vi "Integral.vi"(5 "End":dbl, 7 "Start":dbl, 11 "Spectras-Analiza":cluster{dbl[], dbl[]}[](array[cluster])) -> (3 "Integral":dbl[](array[numeric]))   [LabVIEW 2020]
uses:
  <vilib>/Analysis/2dsp.llb/Integral Method.ctl
  <vilib>/Analysis/8numeric.llb/1D Numeric Integration.vi
  <vilib>/Analysis/NI_AALPro.lvlib
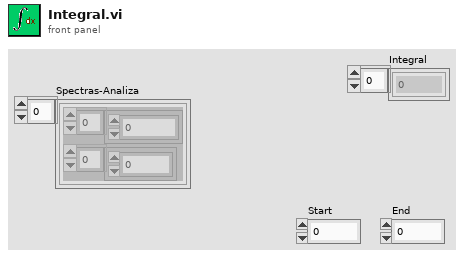
[diagram p1: front panel]
types:
  T1 = typedef "NI_AALPro.lvlib/Integral Method.ctl" = i32
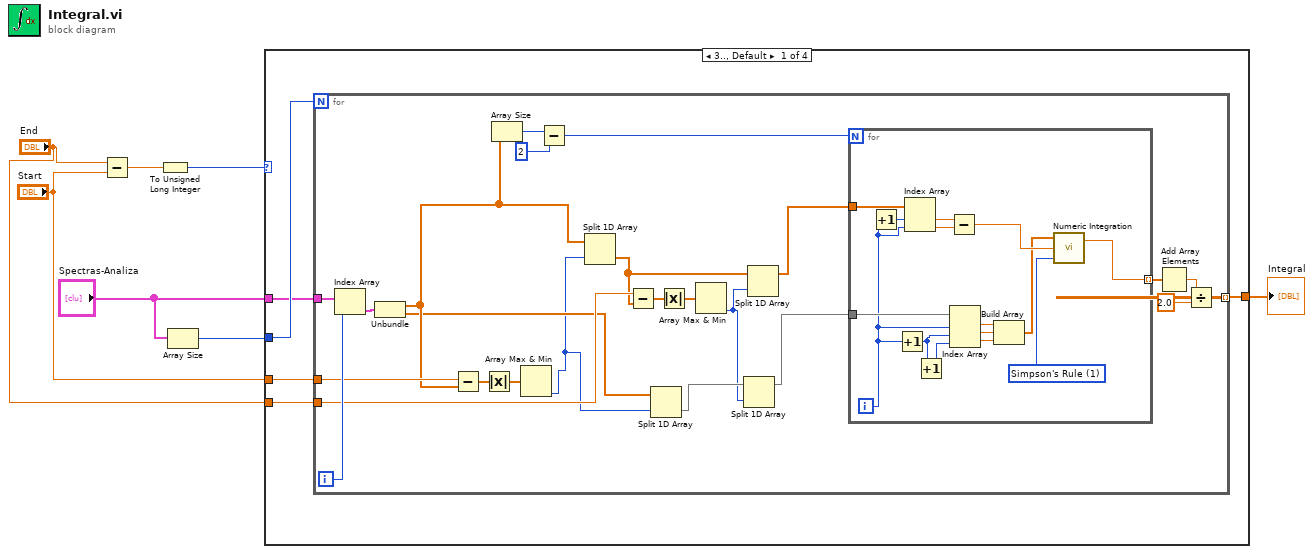
[diagram p0: block diagram]
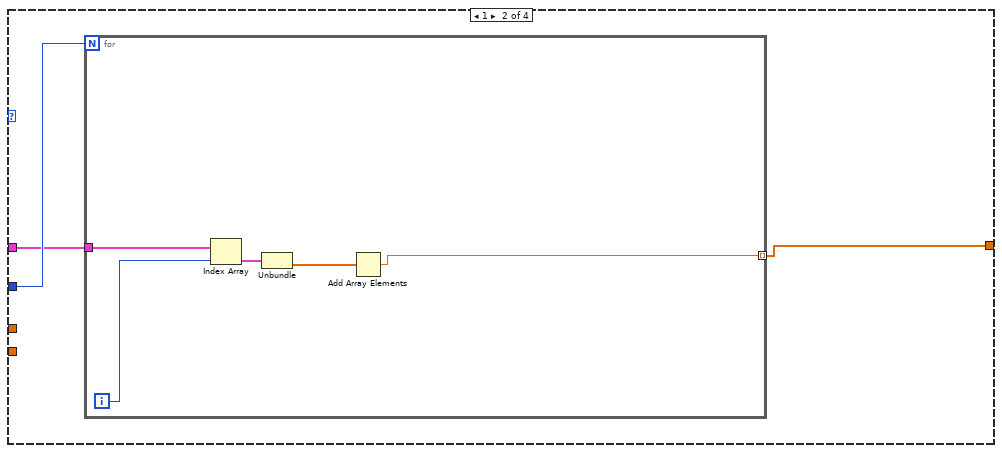
[diagram p2: hidden frame]
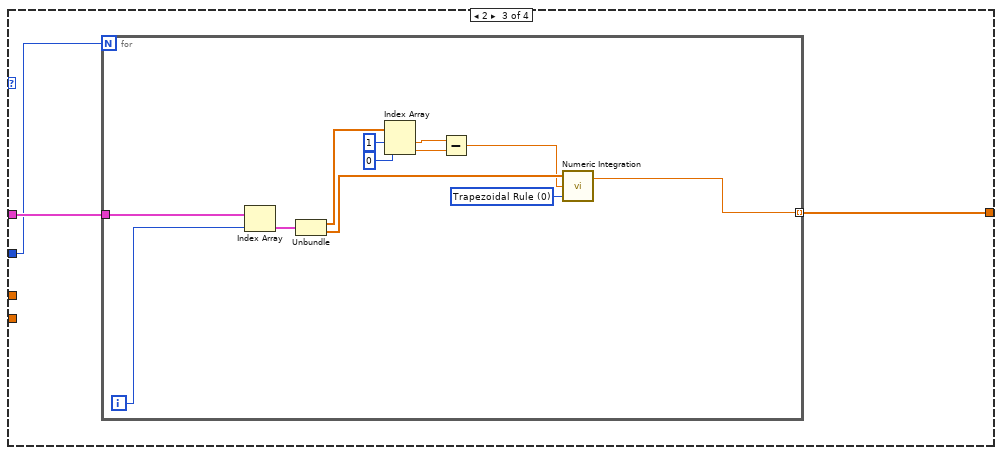
[diagram p3: hidden frame]
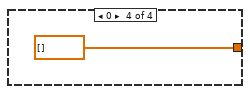
[diagram p4: hidden frame]
diagram:
  n1 = Subtract(x="End", y="Start") -> (x-y=w4:dbl)
  n2 = To Unsigned Long Integer(number=w4) -> (unsigned 32bit integer=w3:u32)
  n3 = Array Size(array="Spectras-Analiza") -> (size(s)=w7:i32)
  n4 = case shown="3.., Default" w3 {
    tunnel: w7 -> [w12 w54 w60 _]
    tunnel: "Spectras-Analiza" -> [w11 w53 w62 _]
    tunnel: [w10 w52 w61 dbl[] []] -> w5
    tunnel: "Start" -> [w9 _ _ _]
    tunnel: "End" -> [w8 _ _ _]
    frame 3.., Default {
      n5 = for {
        N: w12 -> [_]
        tunnel: w11 -> [w36]
        tunnel: [w27] -> w10 mode=indexing
        tunnel: w9 -> [w26]
        tunnel: w8 -> [w22]
        i -> [w35]
        n6 = Index Array(array=w36, index=w35) -> (element=w34:cluster{dbl[], dbl[]})
        n7 = Unbundle(w34) -> (w21:dbl[], w17:dbl[])
        n8 = Subtract(x=w26, y=w21) -> (x-y=w25:dbl[])
        n9 = Absolute Value(x=w25) -> (abs(x)=w24:dbl[])
        n10 = Array Size(array=w21) -> (size(s)=w33:i32)
        n11 = Array Max & Min(array=w24) -> (min index (indices)=w16:i32)  [unwired: 3 out]
        n12 = Subtract(x=w33, y=2) -> (x-y=w31:i32)
        n13 = Split 1D Array(array=w21, index=w16) -> (second subarray=w19:dbl[])  [unwired: 1 out]
        n14 = Subtract(x=w22, y=w19) -> (x-y=w23:dbl[])
        n15 = Split 1D Array(array=w17, index=w16) -> (second subarray=w15:dbl[])  [unwired: 1 out]
        n16 = Absolute Value(x=w23) -> (abs(x)=w20:dbl[])
        n17 = Array Max & Min(array=w20) -> (min index (indices)=w14:i32)  [unwired: 3 out]
        n18 = Split 1D Array(array=w15, index=w14) -> (first subarray=w13:dbl[])  [unwired: 1 out]
        n19 = Split 1D Array(array=w19, index=w14) -> (first subarray=w18:dbl[])  [unwired: 1 out]
        n20 = for {
          N: w31 -> [_]
          tunnel: w18 -> [w50]
          tunnel: w13 -> [w45]
          tunnel: [w37] -> w30 mode=indexing
          i -> [w44]
          w51 = T1 1 items=["Trapezoidal Rule", "Simpson's Rule", "Simpson's 3/8 Rule", "Bode Rule"] ("integration method")
          n21 = Increment(x=w44) -> (x+1=w49:i32)
          n22 = Increment(x=w44) -> (x+1=w42:i32)
          n23 = Index Array(array=w50, index #1=w49, index #2=w44) -> (element #1=w48:dbl, element #2=w47:dbl)
          n24 = Increment(x=w42) -> (x+1=w43:i32)
          n25 = Subtract(x=w48, y=w47) -> (x-y=w46:dbl)
          n26 = Index Array(array=w45, index #1=w44, index #2=w42, index #3=w43) -> (element #1=w41:dbl, element #2=w40:dbl, element #3=w39:dbl)
          n27 = Build Array(w41, w40, w39) -> (w38:dbl[])
          n28 = call-poly <vilib>:"Numeric Integration.vi"("integration method"=w51, "dt"=w46, "Input Array"=w38) -> ("result"=w37:dbl)  [unwired: 1 out]
        }
        n29 = Add Array Elements(numeric array=w30) -> (sum=w29:dbl)
        n30 = Divide(x=w29, y=2.0) -> (x/y=w27:dbl)
      }
    }
    frame 1 {
      n31 = for {
        N: w54 -> [_]
        tunnel: w53 -> [w57]
        tunnel: [w55] -> w52 mode=indexing
        i -> [w58]
        n32 = Index Array(array=w57, index=w58) -> (element=w59:cluster{dbl[], dbl[]})
        n33 = Unbundle(w59) -> (w56:dbl[])  [unwired: 1 out]
        n34 = Add Array Elements(numeric array=w56) -> (sum=w55:dbl)
      }
    }
    frame 2 {
      n35 = for {
        N: w60 -> [_]
        tunnel: w62 -> [w73]
        tunnel: [w63] -> w61 mode=indexing
        i -> [w72]
        w66 = T1 0 items=["Trapezoidal Rule", "Simpson's Rule", "Simpson's 3/8 Rule", "Bode Rule"] ("integration method")
        n36 = Index Array(array=w73, index=w72) -> (element=w74:cluster{dbl[], dbl[]})
        n37 = Unbundle(w74) -> (w71:dbl[], w65:dbl[])
        n38 = Index Array(array=w71, index #1=1 ("index"), index #2=0 ("index")) -> (element #1=w68:dbl, element #2=w67:dbl)
        n39 = Subtract(x=w68, y=w67) -> (x-y=w64:dbl)
        n40 = call-poly <vilib>:"Numeric Integration.vi"("integration method"=w66, "dt"=w64, "Input Array"=w65) -> ("result"=w63:dbl)  [unwired: 1 out]
      }
    }
    frame 0 {
    }
  }
  "Integral" <- w5
